vi "sinEncRanger.vi"(4 "Initial Gains":dbl[](array[numeric])=[1.0, 0.0, 1.0, 0.0, 0.0], 6 "Update skew?":bool=TRUE, 7 "Force No Update":bool, 11 "Cos Sin Input":dbl[](array[numeric])) -> (0 "theta":dbl[](array[numeric]), 3 "Cos Sin Output":dbl[](array[numeric]))   [LabVIEW 2018, in "kevLib2010.lvlib"]
uses:
  kevLib2010.lvlib
panel:
  # "Sin Ranger\nThe purpose of this function is to slowly adapt to adjust for a sinusoids deviation\nfrom a perfect circle.  Given a sine and cosine signal, the function attempts to \noutput the same sine and cosine, but without the offset or gain difference each \nmay have.\n\nNOTE: Try to make the gain as close to 1 as possible before entering.  \nThis affects the learning gain."
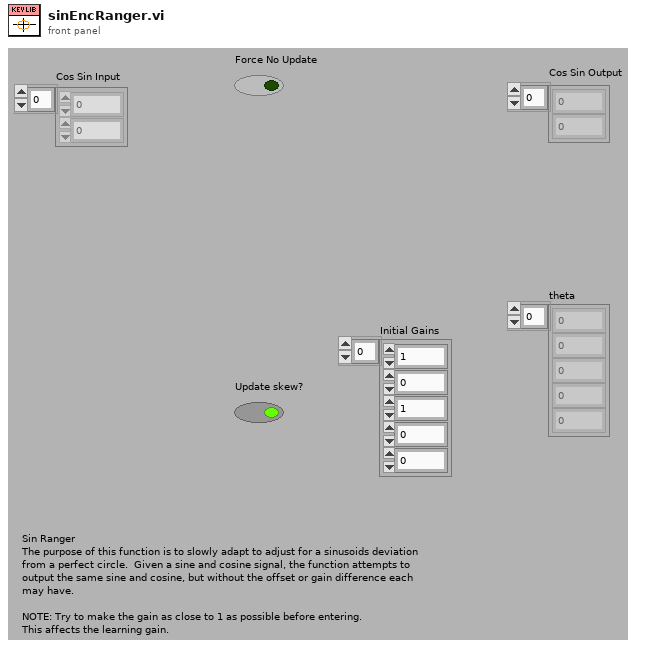
[diagram p1: front panel]
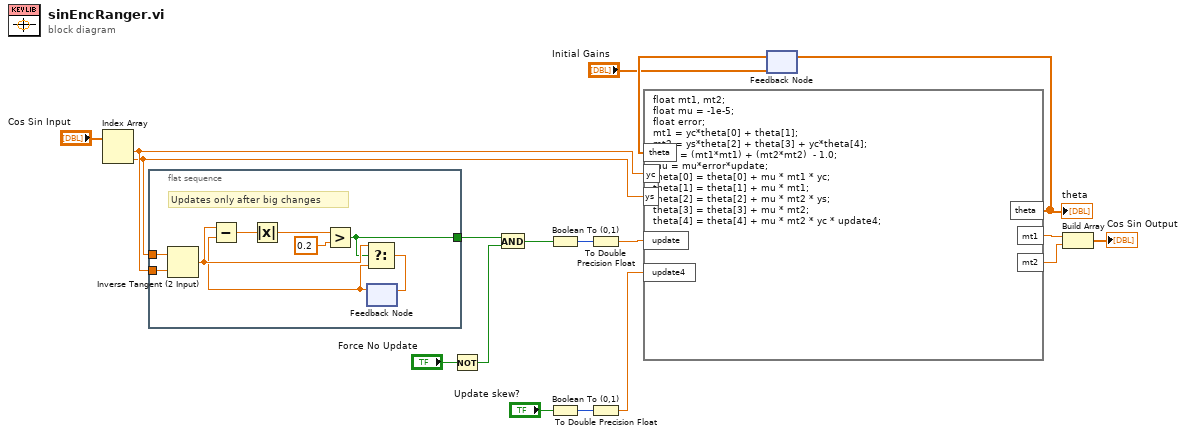
[diagram p0: block diagram]
diagram:
  n1 = Index Array(array="Cos Sin Input") -> (element #1=w8:dbl, element #2=w7:dbl)  [unwired: 2 in]
  n2 = flat-sequence {
    tunnel: w8 -> [w27]
    tunnel: w7 -> [w26]
    tunnel: [w19] -> w13
    frame #0 {
      # "Updates only after big changes"
      n3 = Inverse Tangent (2 Input)(1:w27, 2:w26) -> (0:w25:dbl)
      n4 = feedback #1() -> (w20:dbl)  [unwired: 1 in]
      n5 = Subtract(x=w25, y=w20) -> (x-y=w22:dbl)
      n6 = Absolute Value(x=w22) -> (abs(x)=w21:dbl)
      n7 = Greater?(x=w21, y=0.2) -> (0:w19:bool)
      n8 = Select(t=w25, s=w19, f=w20) -> (s? t:f=w24:dbl)
      n9 = feedback-in #1(w24) -> ()
    }
  }
  n10 = Not(x="Force No Update") -> (.not. x?=w11:bool)
  n11 = And(x=w13, y=w11) -> (x .and. y?=w10:bool)
  n12 = Boolean To (0,1)(Boolean=w10) -> (0, 1=w18:i16)
  n13 = Boolean To (0,1)(Boolean="Update skew?") -> (0, 1=w3:i16)
  n14 = To Double Precision Float(number=w18) -> (double precision float=w17:dbl)
  n15 = To Double Precision Float(number=w3) -> (double precision float=w1:dbl)
  n16 = feedback #2("Initial Gains") -> (w16:dbl[])
  n17 = formula code="float mt1, mt2;\nfloat mu = -1e-5;\nfloat error;\nmt1 = yc*theta[0] + theta[1];\nmt2 = ys*theta[2] + theta[3] + yc*theta[4];\nerror = (mt1*mt1) + (mt2*mt2)  - 1.0;\nmu = mu*error*update;\ntheta[0] = theta[0] + mu * mt1 * yc;\ntheta[1] = theta[1] + mu * mt1;\ntheta[2] = theta[2] + mu * mt2 * ys;\ntheta[3] = theta[3] + mu * mt2;\ntheta[4] = theta[4] + mu * mt2 * yc * update4;"("theta"=w16, "yc"=w8, "ys"=w7, "update"=w17, "update4"=w1) -> ("theta"=w15:dbl[], "mt1"=w6:dbl, "mt2"=w5:dbl)
  "theta" <- w15
  n18 = feedback-in #2(w15) -> ()
  n19 = Build Array(w6, w5) -> (→"Cos Sin Output":dbl[])
